vi "Host - ECAT Slaves write to XML-Log-File.vi"(6 "Operation (0:Öffnen)":T1(ring)=enum."replace or create", 7 "XML Log File name":string="VeriStand_ECAT_Logfile.xml", 8 "Fehler (Eingang, kein Fehler)":errorcluster, 11 "Referenz (Eingang)":refnum<k21>) -> (0 "Fehler (Ausgang)":errorcluster, 2 "Pfad":path, 3 "Referenz (Ausgang)":refnum<k21>)   [LabVIEW 2019, in "SEECD System Explorer.lvlib"]
uses:
  <vilib>/Utility/sysdir.llb/System Directory Type.ctl
  SEECD System Explorer.lvlib
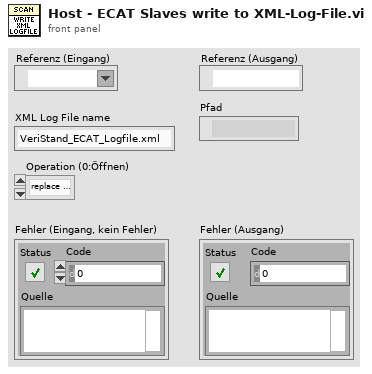
[diagram p1: front panel]
types:
  T1 = enum16{"open", "replace", "create", "open or create", "replace or create", "replace or create with confirmation"}
  T2 = typedef "System Directory Type.ctl" = i32
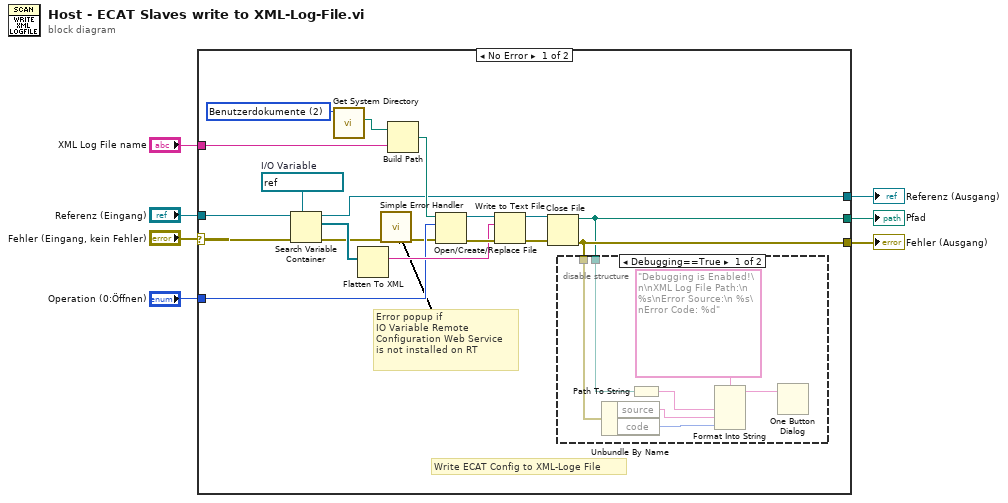
[diagram p0: block diagram]
diagram:
  n1 = case shown="No Error" "Fehler (Eingang, kein Fehler)" {
    selector: "Fehler (Eingang, kein Fehler)" -> [w14 w35]
    tunnel: [w13 w35] -> w7
    tunnel: "Operation (0:Öffnen)" -> [w21 _]
    tunnel: [w19 w34] -> w5
    tunnel: "Referenz (Eingang)" -> [w18 w34]
    tunnel: "XML Log File name" -> [w15 _]
    tunnel: [w12 _] -> w1
    frame No Error {
      w11 = T2 2 items=["Benutzerverzeichnis"=0, "Benutzer-Desktop"=1, "Benutzerdokumente"=2, "Benutzeranwendungsdaten"=3, "Benutzereinstellungen"=4, "Temporäres Verzeichnis"=5, "Öffentliche Dokumente"=6, "Öffentliche Anwendungsdaten"=7, "Öffentliche Einstellungen"=8, "Öffentlicher Cache"=13, "Systembibliotheken"=9, "Installierte Bibliotheken"=10, "Anwendungsdateien"=11, "Boot-Laufwerks-Stammverzeichnis"=12] ("system directory type")
      w17 = refnum<k21> refnum  # I/O Variable
      # "Error popup if\nIO Variable Remote\nConfiguration Web Service\nis not installed on RT"
      # "Write ECAT Config to XML-Loge File"
      n2 = Search Variable Container(7:w17, 8:w14, 11:w18) -> (0:w9:errorcluster, 2:w16:refnum<k21>[], 3:w19:refnum<k21>)  [unwired: 3 in]
      n3 = call <vilib>:"Get System Directory.vi"("system directory type"=w11) -> ("system directory"=w10:path)  [unwired: 10 in]
      n4 = Flatten To XML(anything=w16) -> (xml string=w23:string)
      n5 = call <vilib>:"Simple Error Handler.vi"("error in (no error)"=w9) -> ("error out"=w8:errorcluster)  [unwired: 4 in, 4 out]
      n6 = Build Path(base path=w10, name or relative path=w15) -> (appended path=w20:path)
      n7 = Open/Create/Replace File(file path (use dialog)=w20, error in=w8, operation (0:open)=w21) -> (refnum out=w22:refnum<file>, error out=w24:errorcluster)  [unwired: 3 in, 1 out]
      n8 = Write to Text File(file (use dialog)=w22, text=w23, error in=w24) -> (refnum out=w26:refnum<file>, error out=w25:errorcluster)  [unwired: 1 in, 1 out]
      n9 = Close File(refnum=w26, error in=w25) -> (path=w12:path, error out=w13:errorcluster)
      n10 = disable-structure shown="Debugging==True" {
        disable-tunnel: w13 -> [w33 _]
        disable-tunnel: w12 -> [w32 _]
        frame condition #0 {
          n11 = Unbundle By Name(w33) -> ("source"=w29:string, "code"=w30:i32)
          n12 = Path To String(path=w32) -> (string=w28:string)
          n13 = Format Into String(format string="Debugging is Enabled!\n\nXML Log File Path:\n %s\nError Source:\n %s\nError Code: %d" ("Format-String"), w28, w29, w30) -> (resulting string=w27:string)  [unwired: 2 in, 1 out]
          n14 = One Button Dialog(message=w27) -> ()  [unwired: 1 in, 1 out]
        }
        frame condition #1 (active) {
        }
      }
    }
    frame Error {
    }
  }
  "Fehler (Ausgang)" <- w7
  "Referenz (Ausgang)" <- w5
  "Pfad" <- w1
